vi "Register.vi"(0 "connection reference":T1, 11 "error in (no error)":errorcluster) -> (4 "Patient_ID":i64, 6 "选中个人姓名":string, 8 "选中个人性别":string, 10 "选中个人出生日期":string, 15 "error out":errorcluster)   [LabVIEW 2015, in "Sample.lvlib"]
doc: "使用该模板构建用户界面事件处理设计模式。将模板应用于对话框及其它用户界面。用户也可创建并执行VI可按照与用户界面事件相同方式处理的用户定义事件。"
uses:
  Sample.lvlib
  <vilib>/addons/database/Connection.llb/Conn ObjectReference.ctl
  Support/Register State.ctl
  Support/Register UI State.ctl
  Sub VIs/Database Processing/Database Processing.lvlib
  <vilib>/addons/database/NI_Database_API.lvlib
  Sub VIs/Utility VIs/Utility VIs.lvlib
panel:
  in  "出生日期":string
  in  "性别":string
  in  "姓名":string
  in  "Personal Information":string[][](table)
  in  "Enter":bool caption="New"
  in  "Edit":bool caption="New"
  in  "New":bool
  # "个人资料登记"
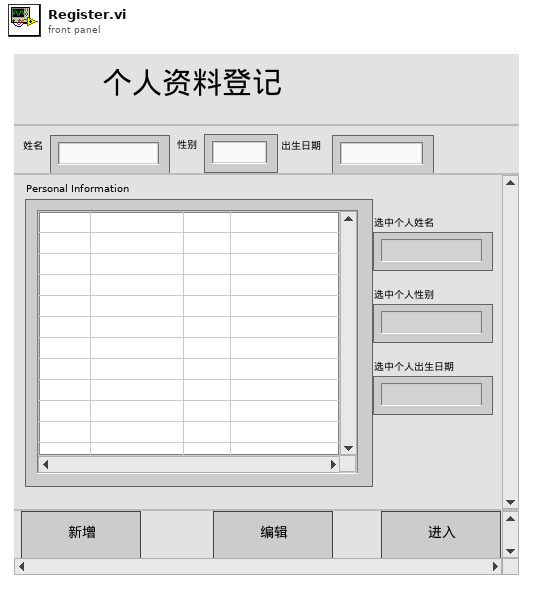
[diagram p1: front panel]
types:
  T1 = typedef "NI_Database_API.lvlib/Conn ObjectReference.ctl" = refnum<k1>
  T2 = typedef "Sample.lvlib/Register UI State.ctl" = cluster{"新增引用句柄":refnum<vi>, "编辑引用句柄":refnum<vi>, "进入引用句柄":refnum<vi>}
  T3 = typedef "Sample.lvlib/Register State.ctl" = enum16{"Initialize", "Connect Database", "Update Personal Information", "Wait For Event", "New", "Edit", "Enter", "Exit", "Update Text Edit"}
  T4 = typedef "Database Processing.lvlib/personal_information.ctl" = cluster{"Patient_ID":i64, "name":string, "sex":string, "birthday":string}
  T5 = typedef "LVPoint32TypeDef.ctl" = cluster{"Horizontal":i32, "Vertical":i32}
  T6 = typedef "LVRowAndColumnTypeDef.ctl" = cluster{"Row":i32, "Column":i32}
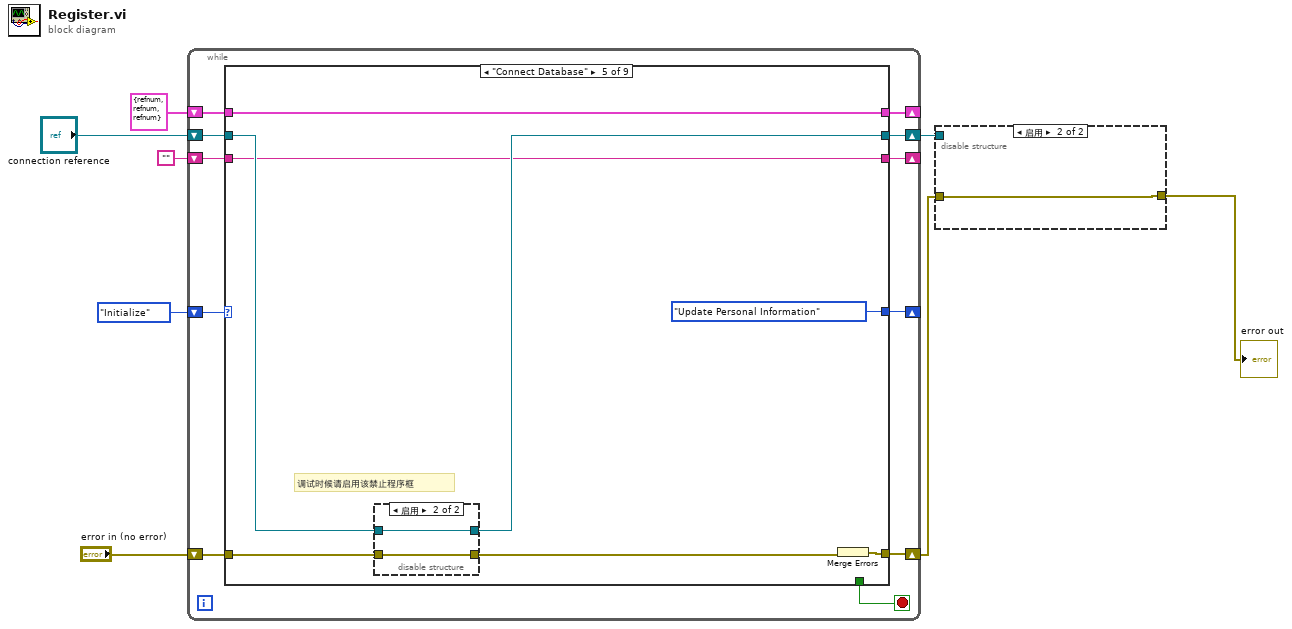
[diagram p0: block diagram]
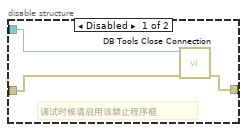
[diagram p2: hidden frame]
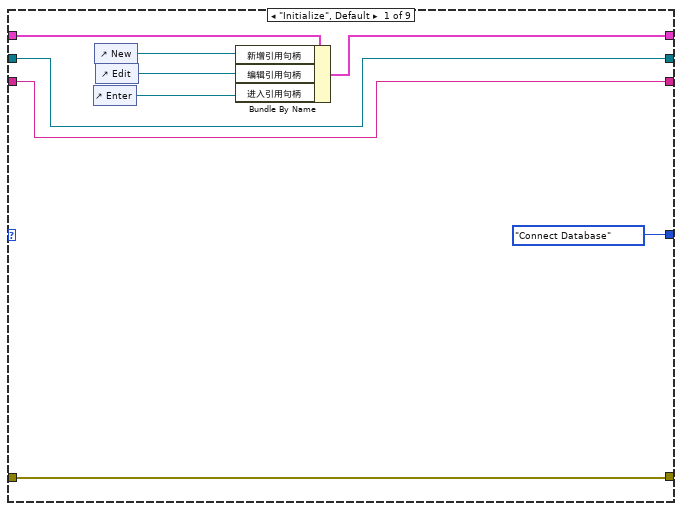
[diagram p3: hidden frame]
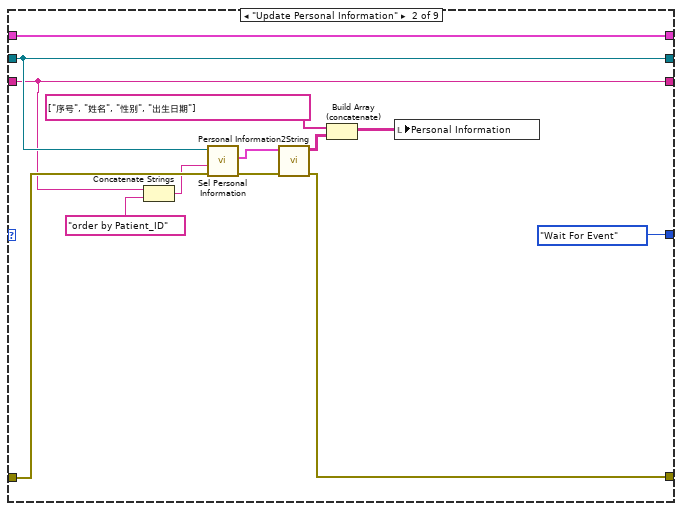
[diagram p4: hidden frame]
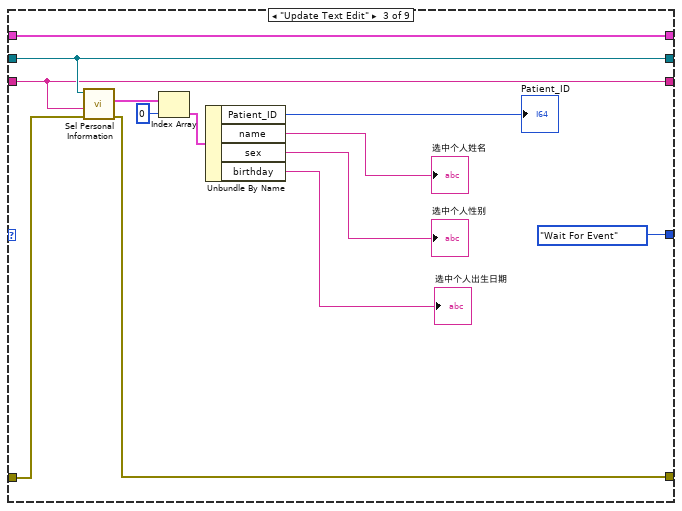
[diagram p5: hidden frame]
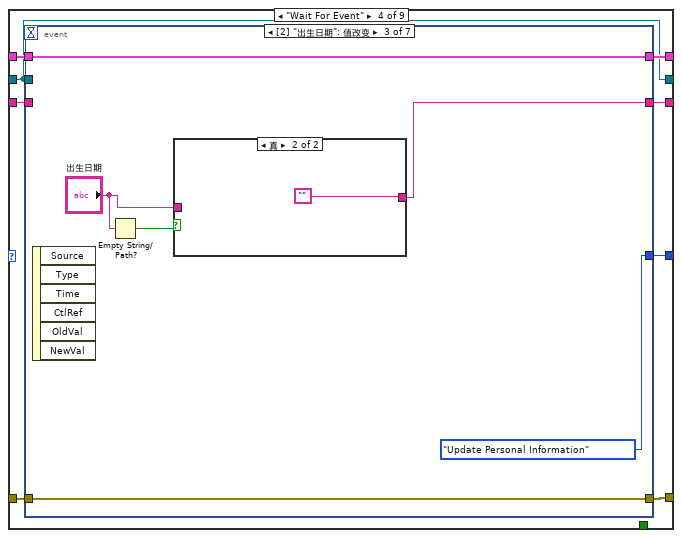
[diagram p6: hidden frame]
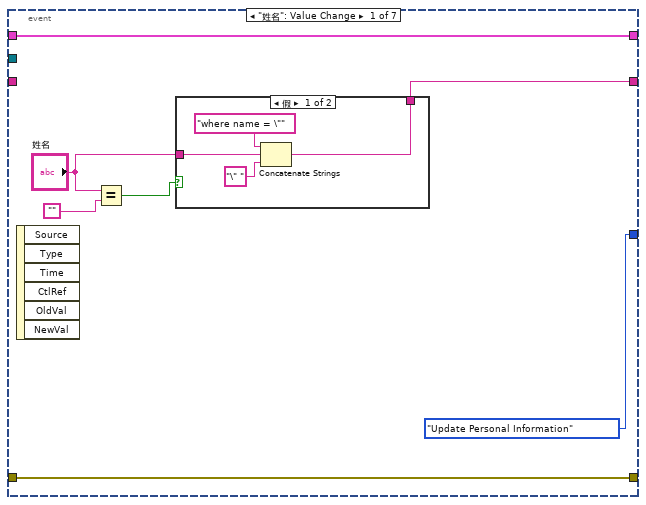
[diagram p7: hidden frame]
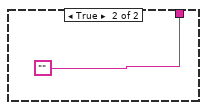
[diagram p8: hidden frame]
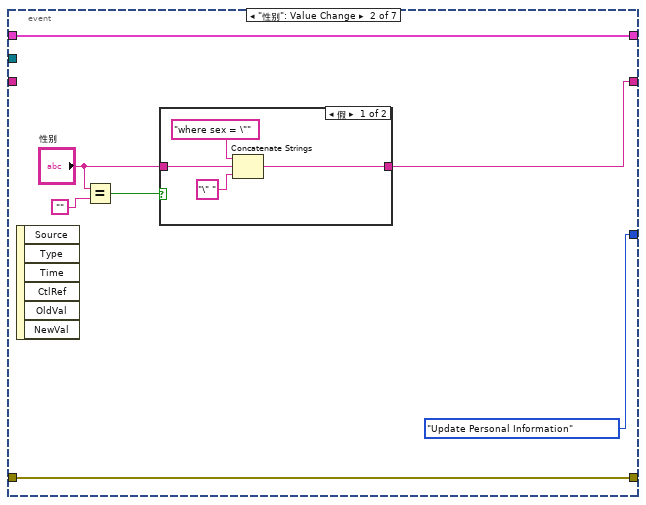
[diagram p9: hidden frame]
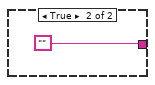
[diagram p10: hidden frame]
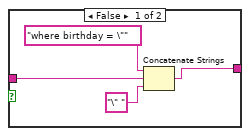
[diagram p11: hidden frame]
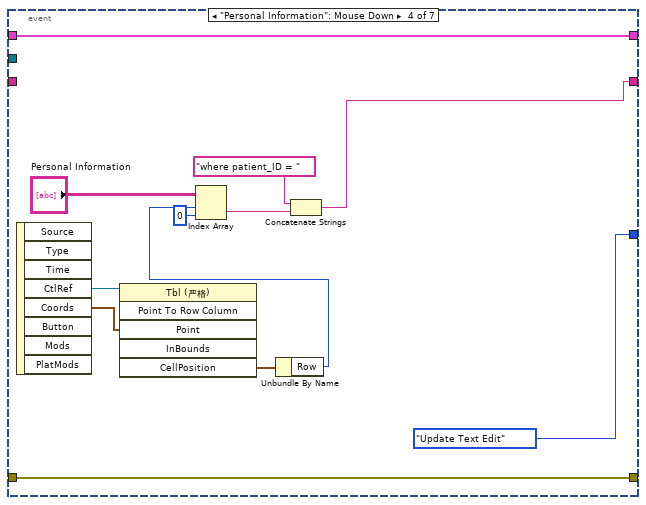
[diagram p12: hidden frame]
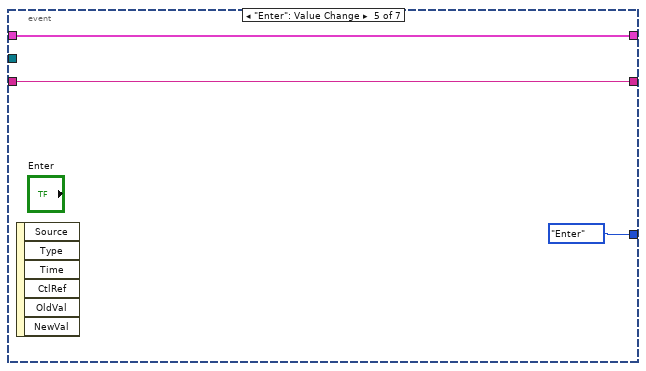
[diagram p13: hidden frame]
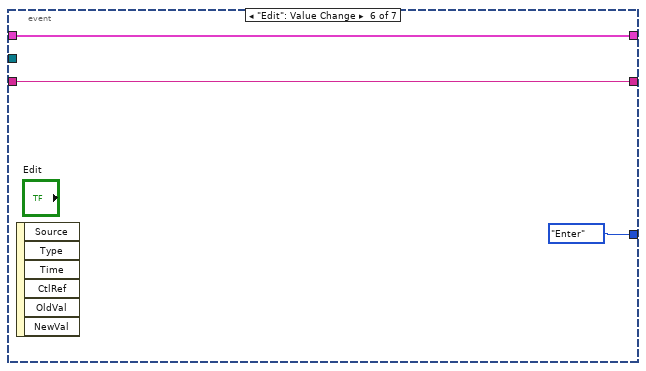
[diagram p14: hidden frame]
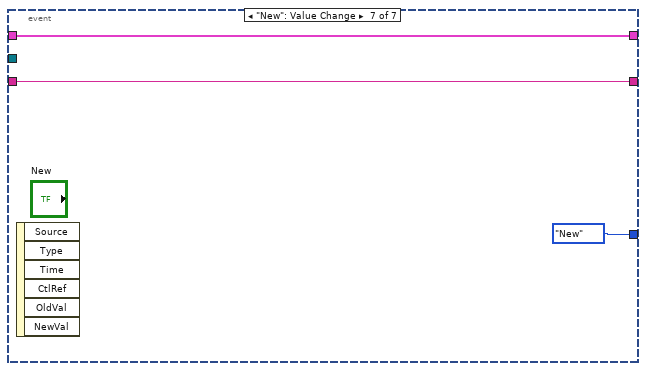
[diagram p15: hidden frame]
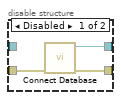
[diagram p16: hidden frame]
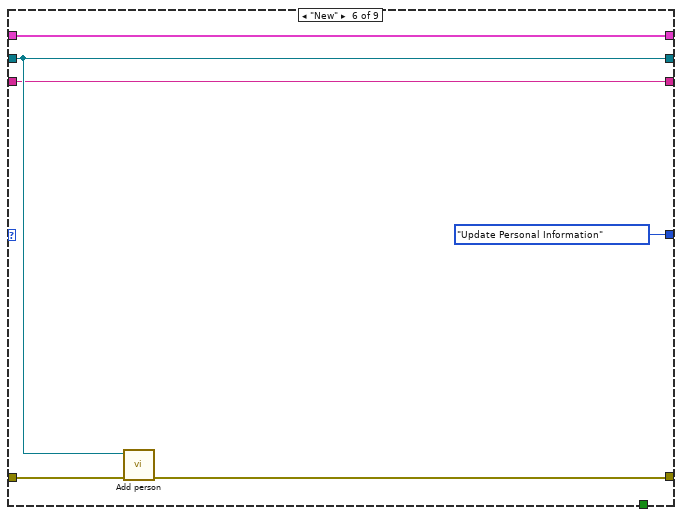
[diagram p17: hidden frame]
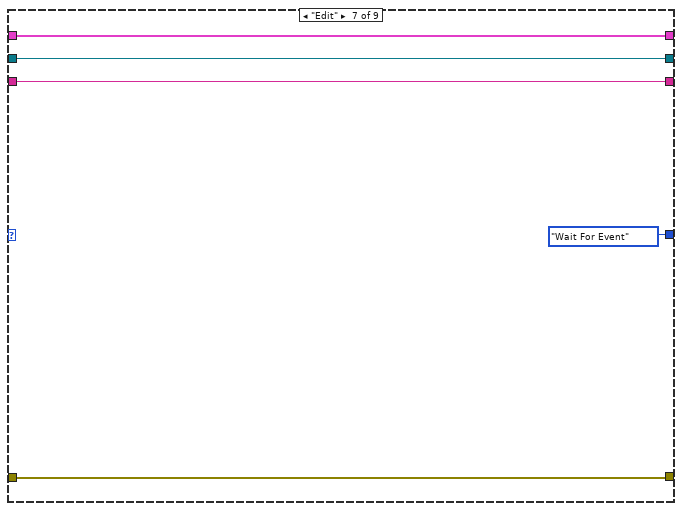
[diagram p18: hidden frame]
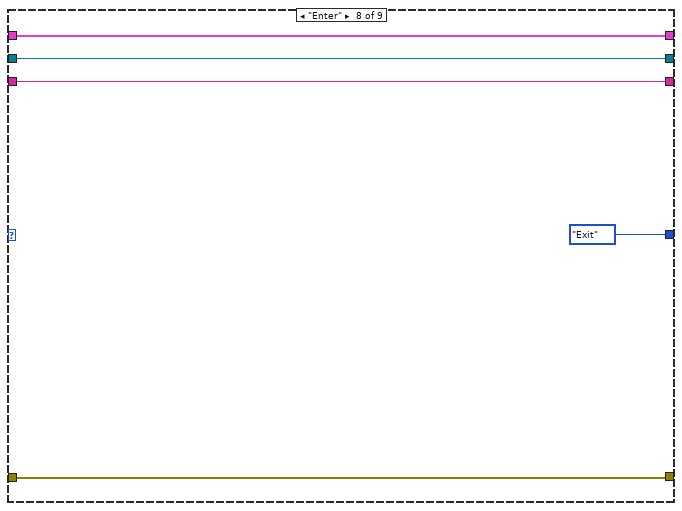
[diagram p19: hidden frame]
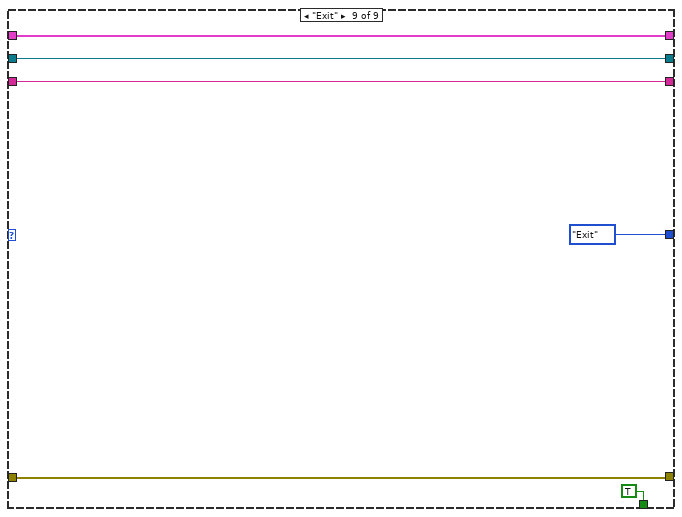
[diagram p20: hidden frame]
diagram:
  n1 = while {
    shift-right: [w17] -> _
    shift-left: T2 {"新增引用句柄"=refnum, "编辑引用句柄"=refnum, "进入引用句柄"=refnum} ("Register UI State") -> [w18]
    shift-right: [w16] -> _
    shift-left: Register_State."Initialize" ("State") -> [w19]
    shift-right: [w14] -> w3
    shift-left: "error in (no error)" -> [w15]
    shift-right: [w12] -> _
    shift-left: "" -> [w13]
    shift-right: [w10] -> w4
    shift-left: "connection reference" -> [w9]
    stop <- w11 stop-if-true
    n2 = case shown="\"Connect Database\"" w19 {
      tunnel: w18 -> [w27 w41 w54 w61 w126 w137 w142 w147 w153]
      tunnel: [w26 w41 w54 w62 w126 w137 w142 w147 w153] -> w17
      tunnel: [Register_State."Connect Database" ("State") Register_State."Wait For Event" ("State") Register_State."Wait For Event" ("State") w60 Register_State."Update Personal Information" ("State") Register_State."Update Personal Information" ("State") Register_State."Wait For Event" ("State") Register_State."Exit" ("State") Register_State."Exit" ("State")] -> w16
      tunnel: w15 -> [w21 w39 w52 w56 w123 w134 w140 w145 w151]
      tunnel: [w21 w33 w51 w57 w124 w133 w140 w145 w151] -> w14
      tunnel: w13 -> [w22 w30 w42 w58 w119 w132 w141 w146 w152]
      tunnel: [w22 w30 w42 w59 w119 w132 w141 w146 w152] -> w12
      tunnel: [_ _ _ _ _ _ _ _ TRUE] -> w11
      tunnel: [w20 w36 w50 w55 w122 w135 w138 w143 w148] -> w10
      tunnel: w9 -> [w20 w36 w50 w55 w121 w135 w138 w143 w148]
      frame "Initialize", Default {
        n3 = control-ref of="Enter"() -> (w23:refnum<vi>)
        n4 = control-ref of="New"() -> (w25:refnum<vi>)
        n5 = control-ref of="Edit"() -> (w24:refnum<vi>)
        n6 = Bundle By Name(cluster=w27, "新增引用句柄"=w25, "编辑引用句柄"=w24, "进入引用句柄"=w23) -> (w26:T2)
      }
      frame "Update Personal Information" {
        n7 = Concatenate Strings(w30, "order by Patient_ID" ("Condition")) -> (w29:string)
        n8 = call "Sel Personal Information.vi"("error in (no error)"=w39, "condition"=w29, "connection reference"=w36) -> ("error out"=w34:errorcluster, "personal information"=w35:T4[])  [unwired: 7 in]
        n9 = call "Personal Information2String.vi"("error in (no error)"=w34, "personal information"=w35) -> ("error out"=w33:errorcluster, "personal information"=w32:string[][])  [unwired: 8 in]
        n10 = Build Array (concatenate)(string[] ["序号", "姓名", "性别", "出生日期"], w32) -> (w37:string[][])
        n11 = local write "Personal Information"(w37) -> ()
      }
      frame "Update Text Edit" {
        n12 = call "Sel Personal Information.vi"("error in (no error)"=w52, "condition"=w42, "connection reference"=w50) -> ("error out"=w51:errorcluster, "personal information"=w49:T4[])  [unwired: 7 in]
        n13 = Index Array(array=w49, index=0 ("索引")) -> (element=w47:T4)
        n14 = Unbundle By Name(w47) -> ("Patient_ID"=→"Patient_ID":i64, "name"=→"选中个人姓名":string, "sex"=→"选中个人性别":string, "birthday"=→"选中个人出生日期":string)
      }
      frame "Wait For Event" {
        n15 = event shown="[2] \"出生日期\": 值改变" {
          selector: _ -> [_ _ _ _ _ _ _]
          dyn-events: _ -> [_ _ _ _ _ _ _]
          timeout: _ -> [_ _ _ _ _ _ _]
          tunnel: [w69 w81 w92 w109 w112 w115 w118] -> w62
          tunnel: w61 -> [w69 w81 w92 w109 w112 w115 w118]
          tunnel: [Register_State."Update Personal Information" ("State") Register_State."Update Personal Information" ("State") Register_State."Update Personal Information" ("State") Register_State."Update Text Edit" ("State") Register_State."Enter" ("State") Register_State."Enter" ("State") Register_State."New" ("State")] -> w60
          tunnel: [w63 w75 w87 w98 w111 w114 w117] -> w59
          tunnel: w58 -> [_ _ _ _ w111 w114 w117]
          tunnel: [w67 w79 w90 w107 _ _ _] -> w57
          tunnel: w56 -> [w67 w79 w90 w107 _ _ _]
          tunnel: w55 -> [_ _ _ _ _ _ _]
          event "姓名": Value Change {
            n16 = event-data() -> ()  [unwired: 1 in, 6 out]
            n17 = Equal?(x="姓名", y="") -> (x = y?=w64:bool)
            n18 = case shown="假" w64 {
              tunnel: [w70 ""] -> w63
              tunnel: "姓名" -> [w71 _]
              frame False {
                n19 = Concatenate Strings("where name = \"", w71, "\" ") -> (w70:string)
              }
              frame True {
              }
            }
          }
          event "性别": Value Change {
            n20 = event-data() -> ()  [unwired: 1 in, 6 out]
            n21 = Equal?(x="性别", y="") -> (x = y?=w76:bool)
            n22 = case shown="假" w76 {
              tunnel: [w82 ""] -> w75
              tunnel: "性别" -> [w83 _]
              frame False {
                n23 = Concatenate Strings("where sex = \"", w83, "\" ") -> (w82:string)
              }
              frame True {
              }
            }
          }
          event "出生日期": Value Change {
            n24 = event-data() -> ()  [unwired: 1 in, 6 out]
            n25 = Empty String/Path?(string/path="出生日期") -> (empty?=w89:bool)
            n26 = case shown="真" w89 {
              tunnel: [w93 ""] -> w87
              tunnel: "出生日期" -> [w94 _]
              frame False {
                n27 = Concatenate Strings("where birthday = \"", w94, "\" ") -> (w93:string)
              }
              frame True {
              }
            }
          }
          event "Personal Information": Mouse Down {
            n28 = event-data() -> ("CtlRef"=w104:refnum<vi>, "Coords"=w106:T5)  [unwired: 1 in, 6 out]
            n29 = invoke class="Tbl (严格)" method="Point To Row Column"(reference=w104, "Point"=w106) -> ("CellPosition"=w105:T6)  [unwired: 4 in, 5 out]
            n30 = Unbundle By Name(w105) -> ("Row"=w102:i32)
            n31 = Index Array(array="Personal Information", index (row)=w102, index (col)=0 ("禁用的索引 (列)")) -> (element=w100:string)
            n32 = Concatenate Strings("where patient_ID = ", w100) -> (w98:string)
          }
          event "Enter": Value Change {
            n33 = event-data() -> ()  [unwired: 1 in, 6 out]
          }
          event "Edit": Value Change {
            n34 = event-data() -> ()  [unwired: 1 in, 6 out]
          }
          event "New": Value Change {
            n35 = event-data() -> ()  [unwired: 1 in, 6 out]
          }
        }
      }
      frame "Connect Database" {
        # "调试时候请启用该禁止程序框"
        n36 = disable-structure shown="启用" {
          disable-tunnel: w123 -> [w129 w131]
          disable-tunnel: [w128 w131] -> w120
          disable-tunnel: [w127 w130] -> w122
          disable-tunnel: w121 -> [_ w130]
          frame Disabled {
            n37 = call "Connect Database.vi"("error in (no error)"=w129) -> ("error out"=w128:errorcluster, "connection reference"=w127:T1)  [unwired: 9 in]
          }
          frame Enabled {
          }
        }
        n38 = Merge Errors(w120) -> (w124:errorcluster)
      }
      frame "New" {
        n39 = call "Add person.vi"("Error In"=w134, "connection reference"=w135) -> ("Error Out"=w133:errorcluster)  [unwired: 8 in, 1 out]
      }
      frame "Edit" {
      }
      frame "Enter" {
      }
      frame "Exit" {
      }
    }
  }
  n40 = disable-structure shown="启用" {
    disable-tunnel: [w156 w157] -> w2
    disable-tunnel: w4 -> [w155 _]
    disable-tunnel: w3 -> [w154 w157]
    frame Disabled {
      # "调试时候请启用该禁止程序框"
      n41 = call <vilib>:"DB Tools Close Connection.vi"("error in (no error)"=w154, "connection reference"=w155) -> ("error out"=w156:errorcluster)  [unwired: 5 in]
    }
    frame Enabled {
    }
  }
  "error out" <- w2
